vi "calc exptime diff.vi"(8 "error in (no error)":errorcluster, 10 "ACS mode":u16(ring), 11 "Simulated_CCD_Camera in":refnum<class "Simulated Camera.lvclass">) -> (0 "error out":errorcluster, 2 "error out":errorcluster, 3 "Simulated_CCD_Camera out":refnum<class "Simulated Camera.lvclass">)   [LabVIEW 2018, in "Simulated Camera.lvclass"]
uses:
  Simulated Camera.lvclass
  Simulated Camera.lvclass/Simulated Camera.ctl
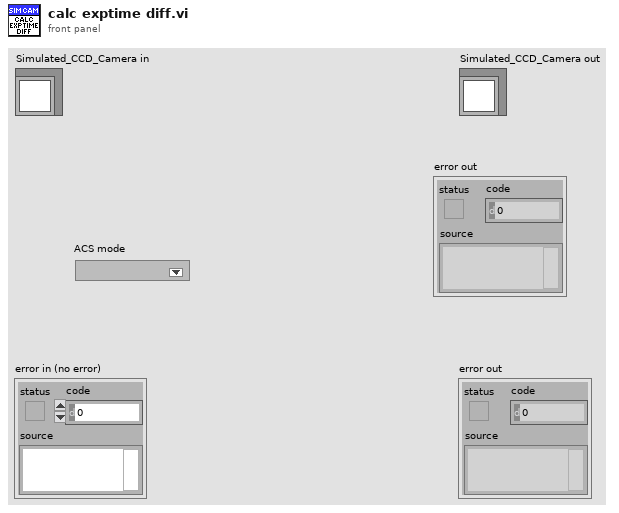
[diagram p1: front panel]
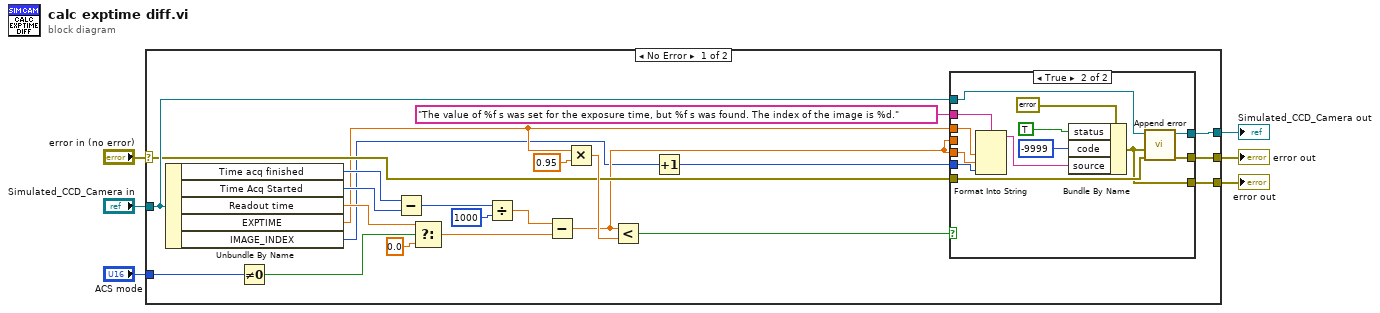
[diagram p0: block diagram]
diagram:
  n1 = case shown="No Error" "error in (no error)" {
    selector: "error in (no error)" -> [w18 w46]
    tunnel: [w16 w46] -> w5
    tunnel: [w17 w45] -> w3
    tunnel: "Simulated_CCD_Camera in" -> [w19 w45]
    tunnel: "ACS mode" -> [w7 _]
    tunnel: [w14 _] -> w1
    frame No Error {
      n2 = Unbundle By Name(w19) -> ("Time acq finished"=w29:u32, "Time Acq Started"=w28:u32, "Readout time"=w22:dbl, "EXPTIME"=w13:dbl, "IMAGE_INDEX"=w10:u32)
      n3 = Not Equal To 0?(x=w7) -> (x != 0?=w8:bool)
      n4 = Subtract(x=w29, y=w28) -> (x-y=w25:u32)
      n5 = Select(t=w22, s=w8, f=0.0) -> (s? t:f=w20:dbl)
      n6 = Divide(x=w25, y=1000) -> (x/y=w23:dbl)
      n7 = Subtract(x=w23, y=w20) -> (x-y=w12:dbl)
      n8 = Multiply(x=w13, y=0.95) -> (x*y=w27:dbl)
      n9 = Less?(x=w12, y=w27) -> (x < y?=w15:bool)
      n10 = Increment(x=w10) -> (x+1=w9:u32)
      n11 = case shown="True" w15 {
        tunnel: w12 -> [_ _]
        tunnel: w19 -> [w30 w39]
        tunnel: w18 -> [w31 w41]
        tunnel: [w30 w38] -> w17
        tunnel: [w31 w40] -> w16
        tunnel: [_ w37] -> w14
        tunnel: w13 -> [_ w36]
        tunnel: w12 -> [_ w35]
        tunnel: "The value of %f s was set for the exposure time, but %f s was found. The index of the image is %d." -> [_ w34]
        tunnel: w9 -> [_ w32]
        frame False {
        }
        frame True {
          n12 = Format Into String(format string=w34, w36, w35, w32) -> (resulting string=w42:string)  [unwired: 2 in, 1 out]
          n13 = Bundle By Name(cluster=errorcluster {"status"=FALSE, "code"=0, "source"=""} ("error out 2"), "status"=TRUE, "code"=-9999, "source"=w42) -> (w37:errorcluster)
          n14 = call "Append error.vi"("error in (no error)"=w41, "error"=w37, "Simulated_CCD_Camera in"=w39) -> ("error out"=w40:errorcluster, "Simulated_CCD_Camera out"=w38:refnum<class "Simulated Camera.lvclass">)  [unwired: 7 in]
        }
      }
    }
    frame Error {
    }
  }
  "error out" <- w5
  "Simulated_CCD_Camera out" <- w3
  "error out" <- w1
